vi "CMD_AEROSCRIPTSTOP.vi"(6 "Gantry in":refnum<class "Gantry.lvclass">, 8 "error in (no error)":errorcluster, 10 "Arguments":string[](array[string]), 11 "gScript Interpreter in":refnum<class "gScript Interpreter.lvclass">) -> (0 "error out":errorcluster, 3 "gScript Interpreter out":refnum<class "gScript Interpreter.lvclass">, 4 "Gantry out":refnum<class "Gantry.lvclass">)   [LabVIEW 2026, in "gScript Interpreter.lvclass"]
uses:
  gScript Interpreter.lvclass
  Shared Components/Gantry Class/Gantry.lvclass
  <instrlib>/Aerotech Automation1/Aerotech Automation1.lvlib
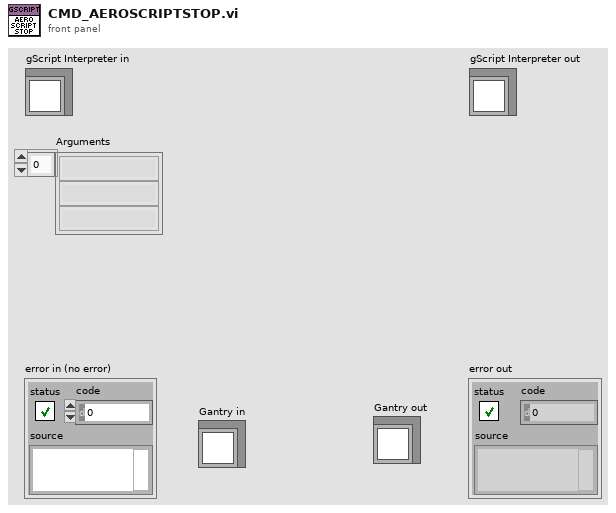
[diagram p1: front panel]
types:
  T1 = enum16{"TLibrary", "T01", "T02", "T03", "T04", "T05", "T06", "T07", "T08", "T09", "T10", "T11", "T12", "T13", "T14", "T15", "T16", "T17", "T18", "T19", "T20", "T21", "T22", "T23", "T24", "T25", "T26", "T27", "T28", "T29", "T30", "T31"}
  T2 = typedef "Virtual Modes.ctl" = enum16{"Nonvirtual", "Virtual"}
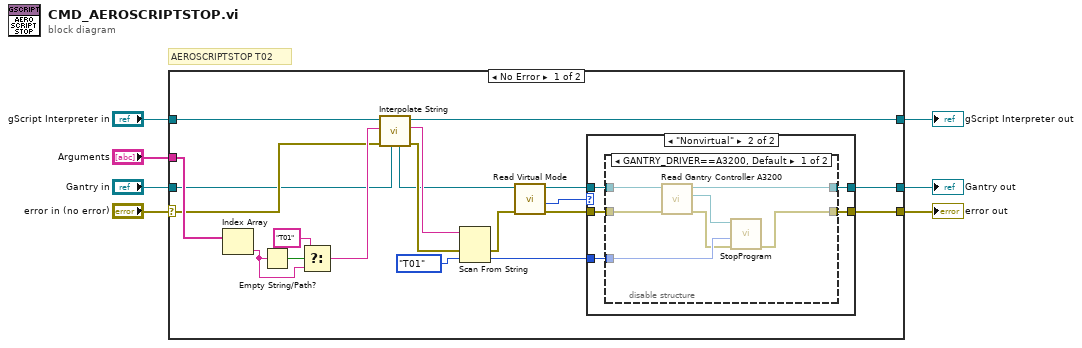
[diagram p0: block diagram]
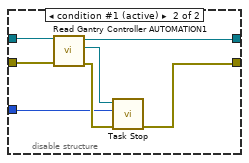
[diagram p3: hidden frame]
diagram:
  # "AEROSCRIPTSTOP T02"
  n1 = case shown="No Error" "error in (no error)" {
    selector: "error in (no error)" -> [w14 w51]
    tunnel: [w26 w51] -> w6
    tunnel: [w17 w50] -> w4
    tunnel: "gScript Interpreter in" -> [w15 w50]
    tunnel: "Arguments" -> [w25 _]
    tunnel: "Gantry in" -> [w13 w49]
    tunnel: [w27 w49] -> w1
    frame No Error {
      n2 = Index Array(array=w25) -> (element=w16:string)  [unwired: 1 in]
      n3 = Empty String/Path?(string/path=w16) -> (empty?=w22:bool)
      n4 = Select(t="T01", s=w22, f=w16) -> (s? t:f=w20:string)
      n5 = call-dynamic "Interpolate String.vi"("Gantry in"=w13, "error in (no error)"=w14, "Input String"=w20, "gScript Interpreter in"=w15) -> ("error out"=w19:errorcluster, "Output String"=w23:string, "gScript Interpreter out"=w17:refnum<class "gScript Interpreter.lvclass">, "Gantry out"=w12:refnum<class "Gantry.lvclass">)  [unwired: 4 in]
      n6 = Scan From String(input string=w23, error in=w19, default 1=T1."T01" ("taskId")) -> (error out=w10:errorcluster, output 1=w18:T1)  [unwired: 2 in, 2 out]
      n7 = call-dynamic "Read Virtual Mode.vi"("error in (no error)"=w10, "Gantry in"=w12) -> ("error out"=w9:errorcluster, "Virtual Mode"=w8:T2, "Gantry out"=w11:refnum<class "Gantry.lvclass">)  [unwired: 6 in, 1 out]
      n8 = case shown="\"Nonvirtual\"" w8 {
        tunnel: w9 -> [w28 w31]
        tunnel: [w29 w30] -> w27
        tunnel: [w28 w34] -> w26
        tunnel: w11 -> [w29 w32]
        tunnel: w18 -> [_ w33]
        frame "Virtual" {
        }
        frame "Nonvirtual" {
          n9 = disable-structure shown="GANTRY_DRIVER==A3200, Default" {
            disable-tunnel: [w41 w42] -> w34
            disable-tunnel: w33 -> [w40 w46]
            disable-tunnel: w32 -> [w39 w45]
            disable-tunnel: w31 -> [w38 w44]
            disable-tunnel: [w35 w43] -> w30
            frame condition #0 {
              n10 = call "Read Gantry Controller A3200.vi"("error in (no error)"=w38, "Gantry in"=w39) -> ("error out"=w37:errorcluster, "A3200 controller out"=w36:refnum<k24>, "Gantry out"=w35:refnum<class "Gantry.lvclass">)  [unwired: 7 in]
              n11 = call "StopProgram.vi"("error in (no error)"=w37, "taskId"=w40, "controller in"=w36) -> ("error out"=w41:errorcluster)  [unwired: 7 in, 1 out]
            }
            frame condition #1 (active) {
              n12 = call "Read Gantry Controller AUTOMATION1.vi"("error in (no error)"=w44, "Gantry in"=w45) -> ("error out"=w47:errorcluster, "Controller AUTOMATION1"=w48:refnum<k24>, "Gantry out"=w43:refnum<class "Gantry.lvclass">)  [unwired: 7 in]
              n13 = call <instrlib>:"Task Stop.vi"("error in (no error)"=w47, "Task Index"=w46, "Controller Refnum"=w48) -> ("error out"=w42:errorcluster)  [unwired: 7 in, 1 out]
            }
          }
        }
      }
    }
    frame Error {
    }
  }
  "error out" <- w6
  "gScript Interpreter out" <- w4
  "Gantry out" <- w1
